vi "Get Fixed & Fitted Parameters v2.vi"(8 "Error In":errorcluster, 9 "Offset Resolution":dbl, 11 "All Parameter Constraints with Values":T1) -> (0 "Error Out":errorcluster, 1 "Fitted Offset":bool, 2 "Offset Array":dbl[](array[numeric]), 3 "Array of Fit Parameter Constraints with Values":T1[](array[typedef]))   [LabVIEW 2021, in "Fits.lvlib"]
uses:
  Fits.lvlib
  IRF(X)PSED/Decay Fit Parameter Constraints with Values.ctl
  IRF(X)PSED/Decay Fit Parameters In List.ctl
  Decay Model.ctl
  Arrays/Linear Ramp End Options.ctl
  Arrays/Arrays.lvlib
  <userlib>/_OpenG.lib/array/array.llb/openg_array.lvlib
  <userlib>/_OpenG.lib/array/array.llb/Sort 1D Array (I16)__ogtk.vi
  <userlib>/_OpenG.lib/array/array.llb/Reorder 1D Array2 (DBL)__ogtk.vi
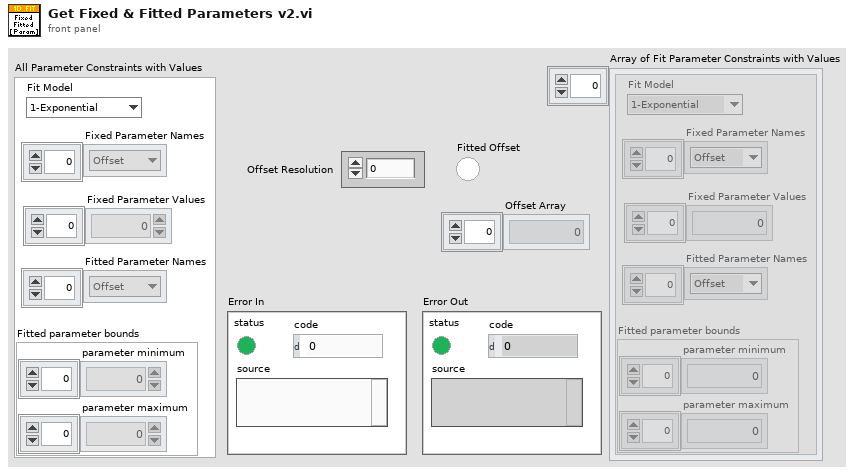
[diagram p1: front panel]
types:
  T1 = typedef "Fits.lvlib/Decay Fit Parameter Constraints with Values.ctl" = cluster{"Fitted parameter bounds":cluster{"parameter minimum":dbl[], "parameter maximum":dbl[]}, "Fixed Parameter Values":dbl[], "Fixed Parameter Names":T2[], "Fitted Parameter Names":T2[], "Fit Model":T3}
  T2 = typedef "Fits.lvlib/Decay Fit Parameters In List.ctl" = enum16{"Offset", "Baseline", "A_1", "tau_1", "A_2", "tau_2"}
  T3 = typedef "Fits.lvlib/Decay Model.ctl" = enum16{"1-Exponential", "2-Exponentials"}
  T4 = typedef "Arrays.lvlib/Linear Ramp End Options.ctl" = enum16{"Include Min/Exclude Max", "Exclude Min/Include Max", "Include Both Ends", "Exclude Both Ends"}
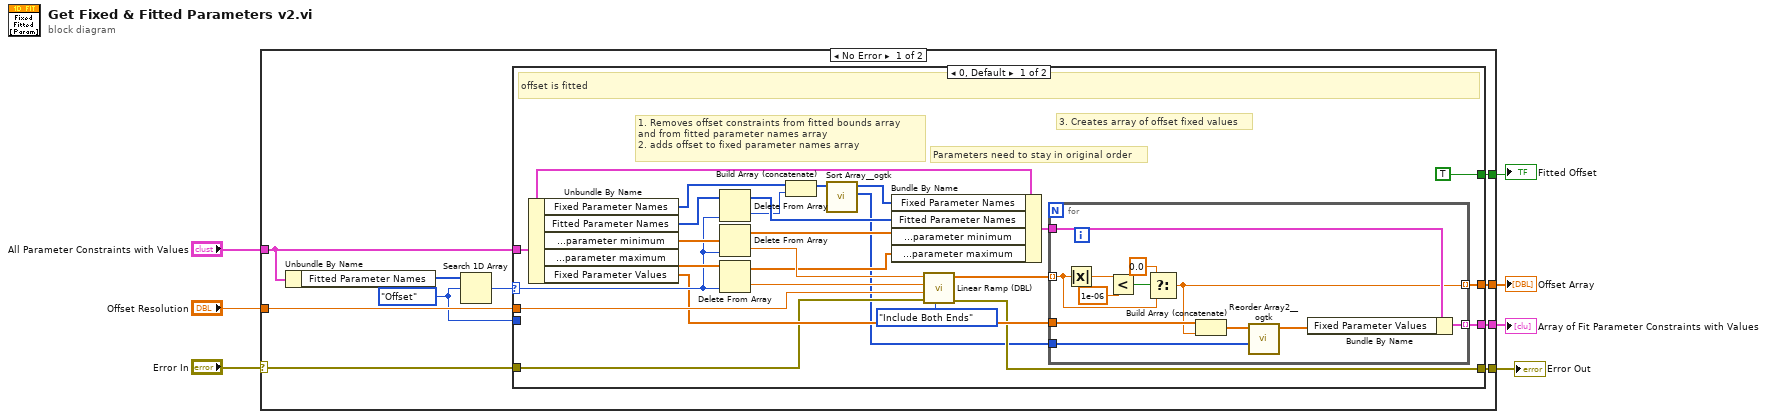
[diagram p0: block diagram]
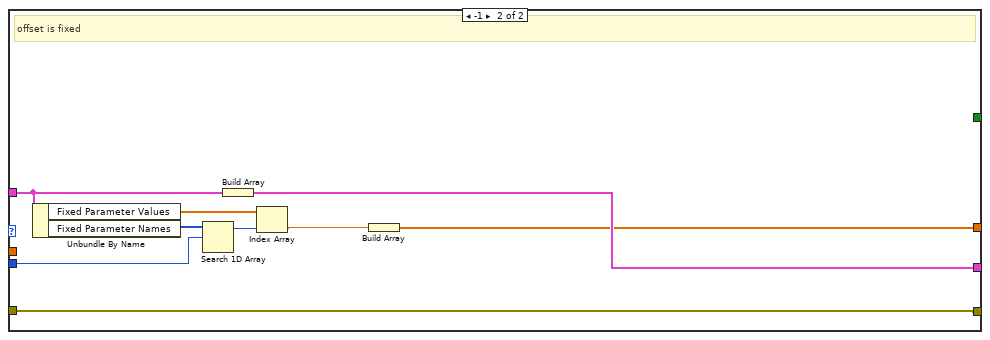
[diagram p2: hidden frame]
diagram:
  n1 = case shown="No Error" "Error In" {
    selector: "Error In" -> [w9 w64]
    tunnel: "All Parameter Constraints with Values" -> [w15 _]
    tunnel: [w14 _] -> w6
    tunnel: "Offset Resolution" -> [w13 _]
    tunnel: [w12 _] -> w4
    tunnel: [w11 _] -> w3
    tunnel: [w8 w64] -> w1
    frame No Error {
      w10 = Decay_Fit_Parameters_In_List."Offset" ("element")
      n2 = Unbundle By Name(w15) -> ("Fitted Parameter Names"=w17:T2[])
      n3 = Search 1D Array(1D array=w17, element=w10) -> (index of element=w16:i32)  [unwired: 1 in]
      n4 = case shown="0, Default" w16 {
        selector: w16 -> [w32 _]
        tunnel: w15 -> [w36 w62]
        tunnel: [w25 w63] -> w14
        tunnel: w13 -> [w38 _]
        tunnel: [TRUE ("Fitted Offset") _] -> w12
        tunnel: [w23 w56] -> w11
        tunnel: w10 -> [_ w60]
        tunnel: w9 -> [w22 w55]
        tunnel: [w21 w55] -> w8
        frame 0, Default {
          # "Parameters need to stay in original order"
          # "Parameters need to stay in original order"
          # "3. Creates array of offset fixed values"
          # "1. Removes offset constraints from fitted bounds array\nand from fitted parameter names array\n2. adds offset to fixed parameter names array"
          # "offset is fitted"
          n5 = Unbundle By Name(w36) -> ("Fixed Parameter Names"=w29:T2[], "Fitted Parameter Names"=w33:T2[], "Fitted parameter bounds.parameter minimum"=w42:dbl[], "Fitted parameter bounds.parameter maximum"=w41:dbl[], "Fixed Parameter Values"=w26:dbl[])
          n6 = Delete From Array(array=w33, index=w32) -> (deleted portion=w30:T2, array with subset deleted=w31:T2[])  [unwired: 1 in]
          n7 = Delete From Array(array=w42, index=w32) -> (deleted portion=w40:dbl, array with subset deleted=w35:dbl[])  [unwired: 1 in]
          n8 = Delete From Array(array=w41, index=w32) -> (deleted portion=w39:dbl, array with subset deleted=w34:dbl[])  [unwired: 1 in]
          n9 = Build Array (concatenate)(w29, w30) -> (w20:T2[])
          n10 = call-poly <userlib>:"Sort Array__ogtk.vi"("Array in"=w20) -> ("Sorted Pointers"=w18:i32[], "Sorted Array out"=w19:i16[])  [unwired: 9 in]
          n11 = Bundle By Name(cluster=w36, "Fixed Parameter Names"=w19, "Fitted Parameter Names"=w31, "Fitted parameter bounds.parameter minimum"=w35, "Fitted parameter bounds.parameter maximum"=w34) -> (w27:T1)
          n12 = call "Linear Ramp (DBL).vi"("Options"=Linear_Ramp_End_Options."Include Both Ends", "Error In"=w22, "Delta"=w38, "Max"=w39, "Min"=w40) -> ("Error Out"=w21:errorcluster, "Ramp"=w28:dbl[])  [unwired: 4 in, 1 out]
          n13 = for {
            tunnel: w28 -> [w46] mode=indexing
            tunnel: w27 -> [w49]
            tunnel: w26 -> [w50]
            tunnel: [w47] -> w25 mode=indexing
            tunnel: [w45] -> w23 mode=indexing
            tunnel: w18 -> [w43]
            n14 = Absolute Value(x=w46) -> (abs(x)=w51:dbl)
            n15 = Less?(x=w51, y=1e-06) -> (x < y?=w53:bool)
            n16 = Select(t=0.0 ("Numeric Control"), s=w53, f=w46) -> (s? t:f=w45:dbl)
            n17 = Build Array (concatenate)(w50, w45) -> (w48:dbl[])
            n18 = call-poly <userlib>:"Reorder Array2__ogtk.vi"("indices"=w43, "array"=w48) -> ("reordered array"=w44:dbl[])  [unwired: 9 in]
            n19 = Bundle By Name(cluster=w49, "Fixed Parameter Values"=w44) -> (w47:T1)
          }
        }
        frame -1 {
          # "offset is fixed"
          n20 = Unbundle By Name(w62) -> ("Fixed Parameter Values"=w59:dbl[], "Fixed Parameter Names"=w61:T2[])
          n21 = Search 1D Array(1D array=w61, element=w60) -> (index of element=w58:i32)  [unwired: 1 in]
          n22 = Build Array(w62) -> (w63:T1[])
          n23 = Index Array(array=w59, index=w58) -> (element=w57:dbl)
          n24 = Build Array(w57) -> (w56:dbl[])
        }
      }
    }
    frame Error {
    }
  }
  "Array of Fit Parameter Constraints with Values" <- w6
  "Error Out" <- w1
  "Fitted Offset" <- w4
  "Offset Array" <- w3
